vi "Scanner.vi"(9 "Continuous":bool, 10 "IntGraph Refnum":refnum<vi>, 11 "Scan Parameters":T1 {"Dwell Time (ms)" min=0; "Y Step" min=0.0; "X Step" min=0.0}) -> (3 "Counts":i32[][](array[numeric]))   [LabVIEW 2012]
uses:
  Strict Type Def - Scan Parameters Cluster.ctl
  <vilib>/DAQmx/write.llb/DAQmx Write (Analog DBL 1Chan 1Samp).vi
  Channels.vi
  <vilib>/DAQmx/create/channels.llb/DAQmx Create Channel (AO-Voltage-Basic).vi
  Global Vars.vi
  <vilib>/DAQmx/miscellaneous.llb/DAQmx Fill In Error Info.vi
panel:
  out "A0 Voltage":dbl caption="A1 Voltage"
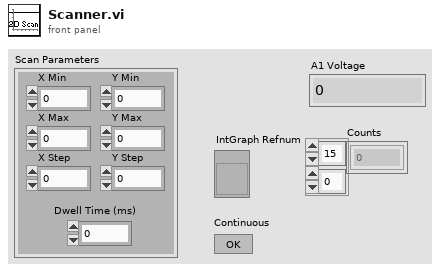
[diagram p1: front panel]
types:
  T1 = typedef "Strict Type Def - Scan Parameters Cluster.ctl" = cluster{"X Max":dbl, "X Min":dbl, "X Step":dbl, "Y Max":dbl, "Y Min":dbl, "Y Step":dbl, "Dwell Time (ms) ":i32}
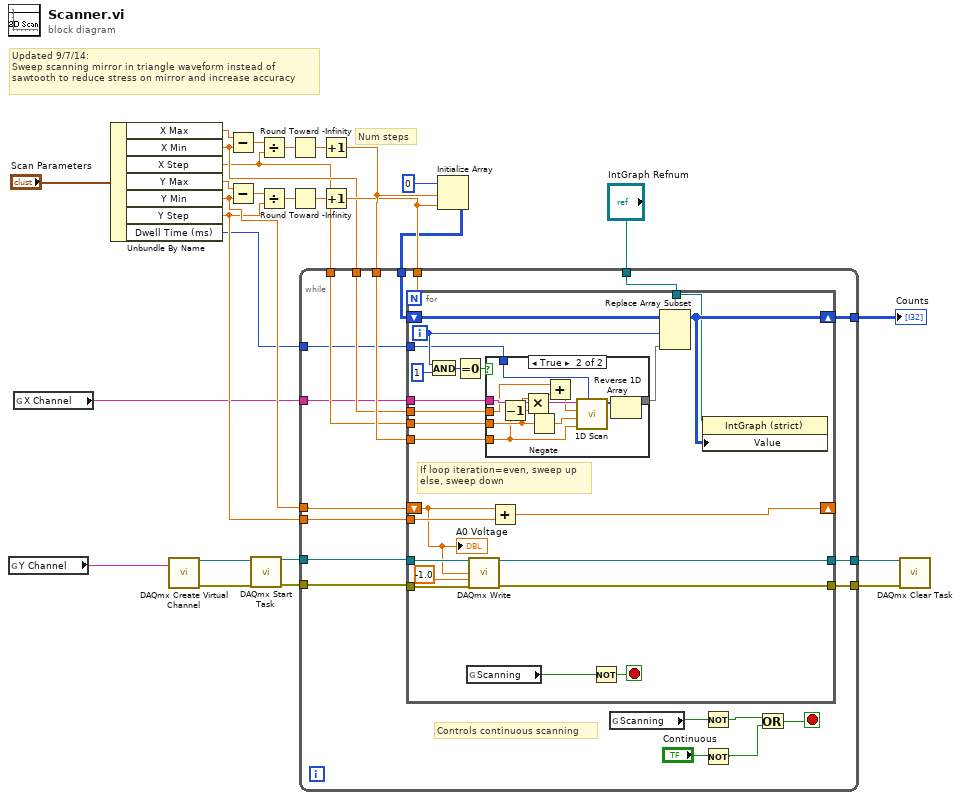
[diagram p0: block diagram]
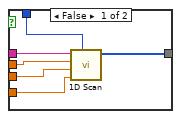
[diagram p2: hidden frame]
diagram:
  # "Num steps"
  # "Updated 9/7/14:\nSweep scanning mirror in triangle waveform instead of\nsawtooth to reduce stress on mirror and increase accuracy"
  n1 = global read "Channels.vi" "Y Channel"() -> (w7:tag)
  n2 = global read "Channels.vi" "X Channel"() -> (w6:tag)
  n3 = Unbundle By Name("Scan Parameters") -> ("X Max"=w1:dbl, "X Min"=w16:dbl, "X Step"=w15:dbl, "Y Max"=w14:dbl, "Y Min"=w13:dbl, "Y Step"=w12:dbl, "Dwell Time (ms)"=w11:i32)
  n4 = call-poly <vilib>:"DAQmx Create Virtual Channel.vi"("physical channels"=w7) -> ("task out"=w5:refnum<k21>, "error out"=w4:errorcluster)  [unwired: 13 in]
  n5 = Subtract(x=w1, y=w16) -> (x-y=w28:dbl)
  n6 = Subtract(x=w14, y=w13) -> (x-y=w27:dbl)
  n7 = call <vilib>:"DAQmx Start Task.vi"("task/channels in"=w5, "error in"=w4) -> ("task out"=w3:refnum<k21>, "error out"=w2:errorcluster)  [unwired: 12 in]
  n8 = Divide(x=w28, y=w15) -> (x/y=w24:dbl)
  n9 = Divide(x=w27, y=w12) -> (x/y=w23:dbl)
  n10 = Round Toward -Infinity(1:w24) -> (0:w21:dbl)
  n11 = Round Toward -Infinity(1:w23) -> (0:w20:dbl)
  n12 = Increment(x=w21) -> (x+1=w19:dbl)
  n13 = Increment(x=w20) -> (x+1=w18:dbl)
  n14 = Initialize Array(u32 0 ("element"), w19, w18) -> (w9:u32[][])
  n15 = while {
    tunnel: [w48] -> w26
    tunnel: [w47] -> w25
    tunnel: w19 -> [w46]
    tunnel: w18 -> [w45]
    tunnel: w16 -> [w44]
    tunnel: w15 -> [w43]
    tunnel: w13 -> [w42]
    tunnel: w12 -> [w41]
    tunnel: w11 -> [w40]
    tunnel: "IntGraph Refnum" -> [w39]
    tunnel: w9 -> [w38]
    tunnel: [w37] -> w8
    tunnel: w6 -> [w36]
    tunnel: w3 -> [w35]
    tunnel: w2 -> [w34]
    stop <- w33 stop-if-true
    # "Controls continuous scanning"
    n16 = for {
      N: w45 -> [_]
      shift-right: [w71] -> _
      shift-left: w42 -> [w64]
      tunnel: [w69] -> w48
      tunnel: [w68] -> w47
      tunnel: w35 -> [w67]
      tunnel: w34 -> [w66]
      tunnel: w44 -> [w59]
      tunnel: w43 -> [w58]
      tunnel: w41 -> [w65]
      tunnel: w46 -> [w57]
      tunnel: w40 -> [w52]
      tunnel: w39 -> [w49]
      tunnel: w36 -> [w50]
      shift-right: [w62] -> w37
      shift-left: w38 -> [w63]
      i -> [w53]
      stop <- w60 stop-if-true
      # "If loop iteration=even, sweep up\nelse, sweep down"
      n17 = And(x=w53, y=u32 1 ("element")) -> (x .and. y?=w54:u32)
      n18 = Equal To 0?(x=w54) -> (x = 0?=w56:bool)
      n19 = global read "Global Vars.vi" "Scanning"() -> (w61:bool)
      n20 = call-poly <vilib>:"DAQmx Write.vi"("task/channels in"=w67, "data"=w64, "timeout"=-1.0, "error in"=w66) -> ("task out"=w69:refnum<k21>, "error out"=w68:errorcluster)  [unwired: 9 in, 1 out]
      n21 = case shown="True" w56 {
        tunnel: w59 -> [w75 w82]
        tunnel: w58 -> [w74 w80]
        tunnel: w57 -> [w73 w79]
        tunnel: w52 -> [w76 w88]
        tunnel: [w77 w84] -> w51
        tunnel: w50 -> [w72 w87]
        frame False {
          n22 = call "1D Scan.vi"("Dwell Time (ms)"=w76, "Num Steps"=w73, "Step"=w74, "Min"=w75, "Channel"=w72) -> ("Counts"=w77:i32[])  [unwired: 6 in]
        }
        frame True {
          n23 = Decrement(x=w79) -> (x-1=w78:dbl)
          n24 = Multiply(x=w80, y=w78) -> (x*y=w83:dbl)
          n25 = Negate(x=w80) -> (-x=w86:dbl)
          n26 = Add(x=w82, y=w83) -> (x+y=w81:dbl)
          n27 = call "1D Scan.vi"("Dwell Time (ms)"=w88, "Num Steps"=w79, "Step"=w86, "Min"=w81, "Channel"=w87) -> ("Counts"=w85:i32[])  [unwired: 6 in]
          n28 = Reverse 1D Array(array=w85) -> (reversed array=w84:i32[])
        }
      }
      n29 = Add(x=w64, y=w65) -> (x+y=w71:dbl)
      n30 = Not(x=w61) -> (.not. x?=w60:bool)
      n31 = Replace Array Subset(array=w63, new element=w51, index (col)=w53) -> (w62:u32[][])  [unwired: 1 in]
      n32 = property class="IntGraph (strict)"(reference=w49, "Value"=w62) -> ()  [unwired: 1 in, 2 out]
      "A0 Voltage" <- w64
    }
    n33 = global read "Global Vars.vi" "Scanning"() -> (w32:bool)
    n34 = Not(x=w32) -> (.not. x?=w31:bool)
    n35 = Not(x="Continuous") -> (.not. x?=w29:bool)
    n36 = Or(x=w31, y=w29) -> (x .or. y?=w33:bool)
  }
  "Counts" <- w8
  n37 = call <vilib>:"DAQmx Clear Task.vi"("task in"=w26, "error in"=w25) -> ()  [unwired: 13 in, 1 out]
